vi "InitializeAllDevices.vi"(8 "error in (no error)":errorcluster, 11 "XML File Name":string) -> (0 "error out":errorcluster, 1 "Meter":refnum<class "Meter.lvclass">, 2 "Scope":refnum<class "Scope.lvclass">, 3 "Signal Generator":refnum<class "Signal Generation.lvclass">, 4 "Switch":refnum<class "Switch.lvclass">)   [LabVIEW 2010]
doc: "InitializeAllDevices first configures the switch to test DUT 1 and then reads the xml configuration file to determine the instrument types, hardware resource names, and DSSP class paths. It then dynamically loads the corresponding DSSP classes and calls the Initialize Device instance of each DSSP class. Each Initialize Device opens the hardware resource session and resets the instrument. \nInitializeAllDevices saves the class references in global variables that are used in the other VIs."
uses:
  DSSP Modules/Output Classes/Signal Generation/Signal Generation.lvclass
  DSSP Modules/Input Classes/Scope/Scope.lvclass
  DSSP Modules/Input Classes/Meter/Meter.lvclass
  DSSP Modules/Output Classes/Switch/Switch.lvclass
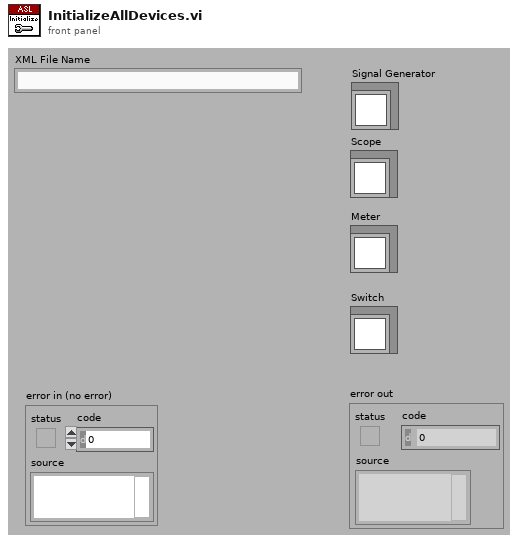
[diagram p1: front panel]
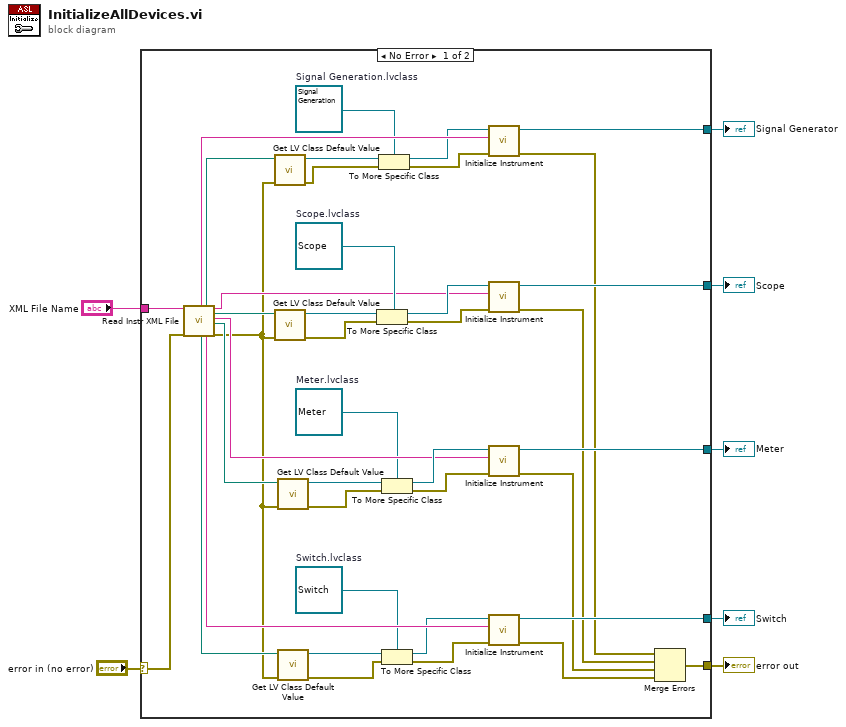
[diagram p0: block diagram]
diagram:
  n1 = case shown="No Error" "error in (no error)" {
    selector: "error in (no error)" -> [w8 w48]
    tunnel: "XML File Name" -> [w35 _]
    tunnel: [w31 _] -> w6
    tunnel: [w30 _] -> w5
    tunnel: [w29 _] -> w4
    tunnel: [w17 w48] -> w3
    tunnel: [w14 _] -> w2
    frame No Error {
      w13 = refnum<class "Meter.lvclass"> refnum  # Meter.lvclass
      w16 = refnum<class "Switch.lvclass"> refnum  # Switch.lvclass
      w28 = refnum<class "Signal Generation.lvclass"> refnum  # Signal Generation.lvclass
      w32 = refnum<class "Scope.lvclass"> refnum  # Scope.lvclass
      n2 = call "Read Instr XML File.vi"("XML File Name"=w35, "error in (no error)"=w8) -> ("Instr 1 Resource Str"=w47:string, "Instr 4 Class Path"=w19:path, "Instr 1 Class Path"=w46:path, "Instr 4 Resource Str"=w20:string, "Instr 2 Resource Str"=w24:string, "Instr 2 Class Path"=w23:path, "Instr 3 Resource Str"=w22:string, "Instr 3 Class Path"=w21:path, "error IO"=w18:errorcluster)  [unwired: 9 out]
      n3 = call <vilib>:"Get LV Class Default Value.vi"("error in (no error)"=w18, "class path"=w46) -> ("error out"=w41:errorcluster, "object"=w45:refnum<class>)  [unwired: 8 out]
      n4 = call <vilib>:"Get LV Class Default Value.vi"("error in (no error)"=w18, "class path"=w23) -> ("error out"=w39:errorcluster, "object"=w44:refnum<class>)  [unwired: 8 out]
      n5 = call <vilib>:"Get LV Class Default Value.vi"("error in (no error)"=w18, "class path"=w21) -> ("error out"=w36:errorcluster, "object"=w37:refnum<class>)  [unwired: 8 out]
      n6 = call <vilib>:"Get LV Class Default Value.vi"("error in (no error)"=w18, "class path"=w19) -> ("error out"=w26:errorcluster, "object"=w25:refnum<class>)  [unwired: 8 out]
      n7 = To More Specific Class(target class=w32, reference=w44, error in=w39) -> (specific class reference=w42:refnum<class "Scope.lvclass">, error out=w38:errorcluster)
      n8 = To More Specific Class(target class=w28, reference=w45, error in=w41) -> (specific class reference=w43:refnum<class "Signal Generation.lvclass">, error out=w40:errorcluster)
      n9 = To More Specific Class(target class=w13, reference=w37, error in=w36) -> (specific class reference=w33:refnum<class "Meter.lvclass">, error out=w34:errorcluster)
      n10 = To More Specific Class(target class=w16, reference=w25, error in=w26) -> (specific class reference=w15:refnum<class "Switch.lvclass">, error out=w27:errorcluster)
      n11 = call-dynamic "Initialize Instrument.vi"("error in (no error)"=w40, "Instr Resource Str"=w47, "DSSP.lvclass in"=w43) -> ("error out"=w12:errorcluster, "DSSP.lvclass out"=w29:refnum<class "Signal Generation.lvclass">)  [unwired: 7 out]
      n12 = call-dynamic "Initialize Instrument.vi"("error in (no error)"=w38, "Instr Resource Str"=w24, "DSSP.lvclass in"=w42) -> ("error out"=w11:errorcluster, "DSSP.lvclass out"=w31:refnum<class "Scope.lvclass">)  [unwired: 7 out]
      n13 = call-dynamic "Initialize Instrument.vi"("error in (no error)"=w34, "Instr Resource Str"=w22, "DSSP.lvclass in"=w33) -> ("error out"=w10:errorcluster, "DSSP.lvclass out"=w30:refnum<class "Meter.lvclass">)  [unwired: 7 out]
      n14 = call-dynamic "Initialize Instrument.vi"("error in (no error)"=w27, "Instr Resource Str"=w20, "DSSP.lvclass in"=w15) -> ("error out"=w9:errorcluster, "DSSP.lvclass out"=w14:refnum<class "Switch.lvclass">)  [unwired: 7 out]
      n15 = Merge Errors(w12, w11, w10, w9) -> (w17:errorcluster)
    }
    frame Error {
    }
  }
  "error out" <- w3
  "Signal Generator" <- w4
  "Scope" <- w6
  "Meter" <- w5
  "Switch" <- w2
